vi "LabVIEW timeout to reqwest timeout.vi"(11 "-1 -> no timeout":i32) -> (3 "0 -> no timeout":u64)   [LabVIEW 2020, in "HTTP Client reqwest.lvclass"]
uses:
  HTTP Client reqwest.lvclass
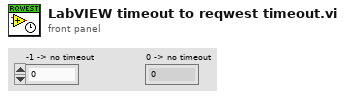
[diagram p1: front panel]
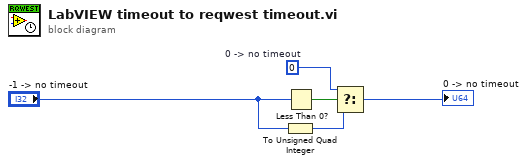
[diagram p0: block diagram]
diagram:
  w1 = u64 0  # 0 -> no timeout
  n1 = To Unsigned Quad Integer(1:"-1 -> no timeout") -> (0:w5:u64)
  n2 = Less Than 0?(x="-1 -> no timeout") -> (x < 0?=w2:bool)
  n3 = Select(t=w1, s=w2, f=w5) -> (s? t:f=→"0 -> no timeout":u64)
